vi "Stop Acquisition.vi"(0 "Stage in":refnum<class "Stage.lvclass">, 1 "Stop":bool, 3 "error in (no error)":errorcluster) -> (7 "Stage out":refnum<class "Stage.lvclass">, 10 "error out":errorcluster)   [LabVIEW 2020, in "Stage.lvlib" / "Stage.lvclass"]
uses:
  Stage.lvclass
  Stage.lvclass/Stage.ctl
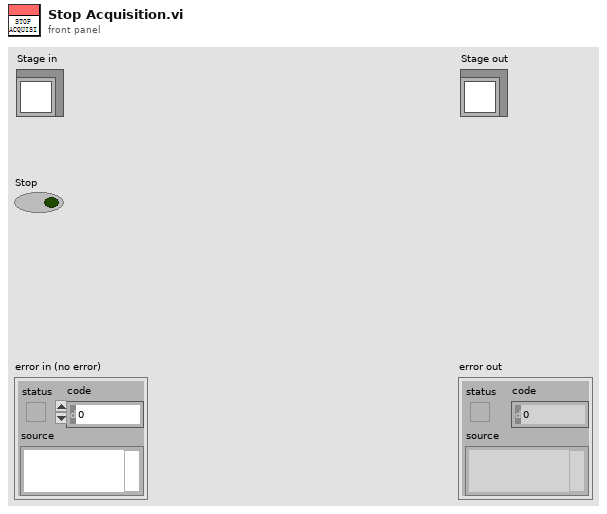
[diagram p1: front panel]
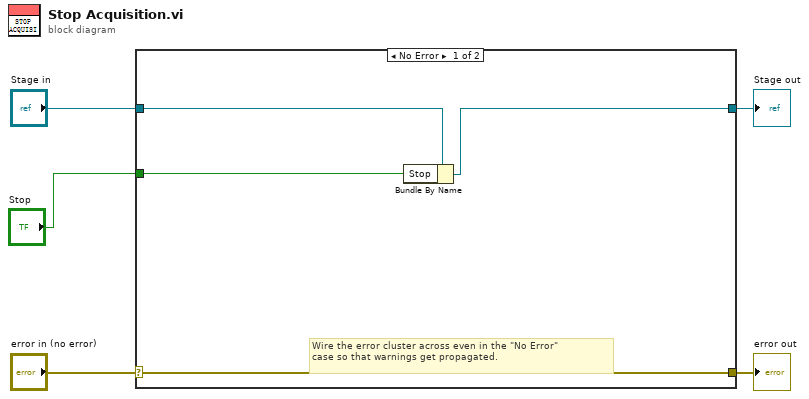
[diagram p0: block diagram]
diagram:
  n1 = case shown="No Error" "error in (no error)" {
    selector: "error in (no error)" -> [w9 w11]
    tunnel: [w9 w11] -> w4
    tunnel: [w6 w10] -> w2
    tunnel: "Stage in" -> [w8 w10]
    tunnel: "Stop" -> [w7 _]
    frame No Error {
      # "Wire the error cluster across even in the \"No Error\"\ncase so that warnings get propagated."
      n2 = Bundle By Name(cluster=w8, "Stop"=w7) -> (w6:refnum<class "Stage.lvclass">)
    }
    frame Error {
    }
  }
  "error out" <- w4
  "Stage out" <- w2
